vi "FipsAdjacent.vi"() -> (11 "Fips":i32[](array[numeric]))   [LabVIEW 2017] (continued)
\t\"Yukon-Koyukuk Census Area, AK\"\t02290\n\"Apache County, AZ\"\t04001\t\"Apache County, AZ\"\t04001\n\"Apache County, AZ\"\t04001\t\"Graham County, AZ\"\t04009\n\"Apache County, AZ\"\t04001\t\"Greenlee County, AZ\"\t04011\n\"Apache County, AZ\"\t04001\t\"Navajo County, AZ\"\t04017\n\"Apache County, AZ\"\t04001\t\"Montezuma County, CO\"\t08083\n\"Apache County, AZ\"\t04001\t\"Catron County, NM\"\t35003\n\"Apache County, AZ\"\t04001\t\"Cibola County, NM\"\t35006\n\"Apache County, AZ\"\t04001\t\"McKinley County, NM\"\t35031\n\"Apache County, AZ\"\t04001\t\"San Juan County, NM\"\t35045\n\"Apache County, AZ\"\t04001\t\"San Juan County, UT\"\t49037\n\"Cochise County, AZ\"\t04003\t\"Cochise County, AZ\"\t04003\n\"Cochise County, AZ\"\t04003\t\"Graham County, AZ\"\t04009\n\"Cochise County, AZ\"\t04003\t\"Greenlee County, AZ\"\t04011\n\"Cochise County, AZ\"\t04003\t\"Pima County, AZ\"\t04019\n\"Cochise County, AZ\"\t04003\t\"Santa Cruz County, AZ\"\t04023\n\"Cochise County, AZ\"\t04003\t\"Hidalgo County, NM\"\t35023\n\"Coconino County, AZ\"\t04005\t\"Coconino County, AZ\"\t04005\n\"Coconino County, AZ\"\t04005\t\"Gila County, AZ\"\t04007\n\"Coconino County, AZ\"\t04005\t\"Mohave County, AZ\"\t04015\n\"Coconino County, AZ\"\t04005\t\"Navajo County, AZ\"\t04017\n\"Coconino County, AZ\"\t04005\t\"Yavapai County, AZ\"\t04025\n\"Coconino County, AZ\"\t04005\t\"Kane County, UT\"\t49025\n\"Coconino County, AZ\"\t04005\t\"San Juan County, UT\"\t49037\n\"Gila County, AZ\"\t04007\t\"Coconino County, AZ\"\t04005\n\"Gila County, AZ\"\t04007\t\"Gila County, AZ\"\t04007\n\"Gila County, AZ\"\t04007\t\"Graham County, AZ\"\t04009\n\"Gila County, AZ\"\t04007\t\"Maricopa County, AZ\"\t04013\n\"Gila County, AZ\"\t04007\t\"Navajo County, AZ\"\t04017\n\"Gila County, AZ\"\t04007\t\"Pinal County, AZ\"\t04021\n\"Gila County, AZ\"\t04007\t\"Yavapai County, AZ\"\t04025\n\"Graham County, AZ\"\t04009\t\"Apache County, AZ\"\t04001\n\"Graham County, AZ\"\t04009\t\"Cochise County, AZ\"\t04003\n\"Graham County, AZ\"\t04009\t\"Gila County, AZ\"\t04007\n\"Graham County, AZ\"\t04009\t\"Graham County, AZ\"\t04009\n\"Graham County, AZ\"\t04009\t\"Greenlee County, AZ\"\t04011\n\"Graham County, AZ\"\t04009\t\"Navajo County, AZ\"\t04017\n\"Graham County, AZ\"\t04009\t\"Pima County, AZ\"\t04019\n\"Graham County, AZ\"\t04009\t\"Pinal County, AZ\"\t04021\n\"Greenlee County, AZ\"\t04011\t\"Apache County, AZ\"\t04001\n\"Greenlee County, AZ\"\t04011\t\"Cochise County, AZ\"\t04003\n\"Greenlee County, AZ\"\t04011\t\"Graham County, AZ\"\t04009\n\"Greenlee County, AZ\"\t04011\t\"Greenlee County, AZ\"\t04011\n\"Greenlee County, AZ\"\t04011\t\"Catron County, NM\"\t35003\n\"Greenlee County, AZ\"\t04011\t\"Grant County, NM\"\t35017\n\"Greenlee County, AZ\"\t04011\t\"Hidalgo County, NM\"\t35023\n\"La Paz County, AZ\"\t04012\t\"La Paz County, AZ\"\t04012\n\"La Paz County, AZ\"\t04012\t\"Maricopa County, AZ\"\t04013\n\"La Paz County, AZ\"\t04012\t\"Mohave County, AZ\"\t04015\n\"La Paz County, AZ\"\t04012\t\"Yavapai County, AZ\"\t04025\n\"La Paz County, AZ\"\t04012\t\"Yuma County, AZ\"\t04027\n\"La Paz County, AZ\"\t04012\t\"Imperial County, CA\"\t06025\n\"La Paz County, AZ\"\t04012\t\"Riverside County, CA\"\t06065\n\"La Paz County, AZ\"\t04012\t\"San Bernardino County, CA\"\t06071\n\"Maricopa County, AZ\"\t04013\t\"Gila County, AZ\"\t04007\n\"Maricopa County, AZ\"\t04013\t\"La Paz County, AZ\"\t04012\n\"Maricopa County, AZ\"\t04013\t\"Maricopa County, AZ\"\t04013\n\"Maricopa County, AZ\"\t04013\t\"Pima County, AZ\"\t04019\n\"Maricopa County, AZ\"\t04013\t\"Pinal County, AZ\"\t04021\n\"Maricopa County, AZ\"\t04013\t\"Yavapai County, AZ\"\t04025\n\"Maricopa County, AZ\"\t04013\t\"Yuma County, AZ\"\t04027\n\"Mohave County, AZ\"\t04015\t\"Coconino County, AZ\"\t04005\n\"Mohave County, AZ\"\t04015\t\"La Paz County, AZ\"\t04012\n\"Mohave County, AZ\"\t04015\t\"Mohave County, AZ\"\t04015\n\"Mohave County, AZ\"\t04015\t\"Yavapai County, AZ\"\t04025\n\"Mohave County, AZ\"\t04015\t\"San Bernardino County, CA\"\t06071\n\"Mohave County, AZ\"\t04015\t\"Clark County, NV\"\t32003\n\"Mohave County, AZ\"\t04015\t\"Lincoln County, NV\"\t32017\n\"Mohave County, AZ\"\t04015\t\"Kane County, UT\"\t49025\n\"Mohave County, AZ\"\t04015\t\"Washington County, UT\"\t49053\n\"Navajo County, AZ\"\t04017\t\"Apache County, AZ\"\t04001\n\"Navajo County, AZ\"\t04017\t\"Coconino County, AZ\"\t04005\n\"Navajo County, AZ\"\t04017\t\"Gila County, AZ\"\t04007\n\"Navajo County, AZ\"\t04017\t\"Graham County, AZ\"\t04009\n\"Navajo County, AZ\"\t04017\t\"Navajo County, AZ\"\t04017\n\"Navajo County, AZ\"\t04017\t\"San Juan County, UT\"\t49037\n\"Pima County, AZ\"\t04019\t\"Cochise County, AZ\"\t04003\n\"Pima County, AZ\"\t04019\t\"Graham County, AZ\"\t04009\n\"Pima County, AZ\"\t04019\t\"Maricopa County, AZ\"\t04013\n\"Pima County, AZ\"\t04019\t\"Pima County, AZ\"\t04019\n\"Pima County, AZ\"\t04019\t\"Pinal County, AZ\"\t04021\n\"Pima County, AZ\"\t04019\t\"Santa Cruz County, AZ\"\t04023\n\"Pima County, AZ\"\t04019\t\"Yuma County, AZ\"\t04027\n\"Pinal County, AZ\"\t04021\t\"Gila County, AZ\"\t04007\n\"Pinal County, AZ\"\t04021\t\"Graham County, AZ\"\t04009\n\"Pinal County, AZ\"\t04021\t\"Maricopa County, AZ\"\t04013\n\"Pinal County, AZ\"\t04021\t\"Pima County, AZ\"\t04019\n\"Pinal County, AZ\"\t04021\t\"Pinal County, AZ\"\t04021\n\"Santa Cruz County, AZ\"\t04023\t\"Cochise County, AZ\"\t04003\n\"Santa Cruz County, AZ\"\t04023\t\"Pima County, AZ\"\t04019\n\"Santa Cruz County, AZ\"\t04023\t\"Santa Cruz County, AZ\"\t04023\n\"Yavapai County, AZ\"\t04025\t\"Coconino County, AZ\"\t04005\n\"Yavapai County, AZ\"\t04025\t\"Gila County, AZ\"\t04007\n\"Yavapai County, AZ\"\t04025\t\"La Paz County, AZ\"\t04012\n\"Yavapai County, AZ\"\t04025\t\"Maricopa County, AZ\"\t04013\n\"Yavapai County, AZ\"\t04025\t\"Mohave County, AZ\"\t04015\n\"Yavapai County, AZ\"\t04025\t\"Yavapai County, AZ\"\t04025\n\"Yuma County, AZ\"\t04027\t\"La Paz County, AZ\"\t04012\n\"Yuma County, AZ\"\t04027\t\"Maricopa County, AZ\"\t04013\n\"Yuma County, AZ\"\t04027\t\"Pima County, AZ\"\t04019\n\"Yuma County, AZ\"\t04027\t\"Yuma County, AZ\"\t04027\n\"Yuma County, AZ\"\t04027\t\"Imperial County, CA\"\t06025\n\"Arkansas County, AR\"\t05001\t\"Arkansas County, AR\"\t05001\n\"Arkansas County, AR\"\t05001\t\"Desha County, AR\"\t05041\n\"Arkansas County, AR\"\t05001\t\"Jefferson County, AR\"\t05069\n\"Arkansas County, AR\"\t05001\t\"Lincoln County, AR\"\t05079\n\"Arkansas County, AR\"\t05001\t\"Lonoke County, AR\"\t05085\n\"Arkansas County, AR\"\t05001\t\"Monroe County, AR\"\t05095\n\"Arkansas County, AR\"\t05001\t\"Phillips County, AR\"\t05107\n\"Arkansas County, AR\"\t05001\t\"Prairie County, AR\"\t05117\n\"Ashley County, AR\"\t05003\t\"Ashley County, AR\"\t05003\n\"Ashley County, AR\"\t05003\t\"Bradley County, AR\"\t05011\n\"Ashley County, AR\"\t05003\t\"Chicot County, AR\"\t05017\n\"Ashley County, AR\"\t05003\t\"Drew County, AR\"\t05043\n\"Ashley County, AR\"\t05003\t\"Union County, AR\"\t05139\n\"Ashley County, AR\"\t05003\t\"Morehouse Parish, LA\"\t22067\n\"Ashley County, AR\"\t05003\t\"Union Parish, LA\"\t22111\n\"Baxter County, AR\"\t05005\t\"Baxter County, AR\"\t05005\n\"Baxter County, AR\"\t05005\t\"Fulton County, AR\"\t05049\n\"Baxter County, AR\"\t05005\t\"Izard County, AR\"\t05065\n\"Baxter County, AR\"\t05005\t\"Marion County, AR\"\t05089\n\"Baxter County, AR\"\t05005\t\"Searcy County, AR\"\t05129\n\"Baxter County, AR\"\t05005\t\"Stone County, AR\"\t05137\n\"Baxter County, AR\"\t05005\t\"Ozark County, MO\"\t29153\n\"Benton County, AR\"\t05007\t\"Benton County, AR\"\t05007\n\"Benton County, AR\"\t05007\t\"Carroll County, AR\"\t05015\n\"Benton County, AR\"\t05007\t\"Madison County, AR\"\t05087\n\"Benton County, AR\"\t05007\t\"Washington County, AR\"\t05143\n\"Benton County, AR\"\t05007\t\"Barry County, MO\"\t29009\n\"Benton County, AR\"\t05007\t\"McDonald County, MO\"\t29119\n\"Benton County, AR\"\t05007\t\"Adair County, OK\"\t40001\n\"Benton County, AR\"\t05007\t\"Delaware County, OK\"\t40041\n\"Boone County, AR\"\t05009\t\"Boone County, AR\"\t05009\n\"Boone County, AR\"\t05009\t\"Carroll County, AR\"\t05015\n\"Boone County, AR\"\t05009\t\"Marion County, AR\"\t05089\n\"Boone County, AR\"\t05009\t\"Newton County, AR\"\t05101\n\"Boone County, AR\"\t05009\t\"Searcy County, AR\"\t05129\n\"Boone County, AR\"\t05009\t\"Taney County, MO\"\t29213\n\"Bradley County, AR\"\t05011\t\"Ashley County, AR\"\t05003\n\"Bradley County, AR\"\t05011\t\"Bradley County, AR\"\t05011\n\"Bradley County, AR\"\t05011\t\"Calhoun County, AR\"\t05013\n\"Bradley County, AR\"\t05011\t\"Cleveland County, AR\"\t05025\n\"Bradley County, AR\"\t05011\t\"Drew County, AR\"\t05043\n\"Bradley County, AR\"\t05011\t\"Union County, AR\"\t05139\n\"Calhoun County, AR\"\t05013\t\"Bradley County, AR\"\t05011\n\"Calhoun County, AR\"\t05013\t\"Calhoun County, AR\"\t05013\n\"Calhoun County, AR\"\t05013\t\"Cleveland County, AR\"\t05025\n\"Calhoun County, AR\"\t05013\t\"Dallas County, AR\"\t05039\n\"Calhoun County, AR\"\t05013\t\"Ouachita County, AR\"\t05103\n\"Calhoun County, AR\"\t05013\t\"Union County, AR\"\t05139\n\"Carroll County, AR\"\t05015\t\"Benton County, AR\"\t05007\n\"Carroll County, AR\"\t05015\t\"Boone County, AR\"\t05009\n\"Carroll County, AR\"\t05015\t\"Carroll County, AR\"\t05015\n\"Carroll County, AR\"\t05015\t\"Madison County, AR\"\t05087\n\"Carroll County, AR\"\t05015\t\"Newton County, AR\"\t05101\n\"Carroll County, AR\"\t05015\t\"Barry County, MO\"\t29009\n\"Carroll County, AR\"\t05015\t\"Stone County, MO\"\t29209\n\"Carroll County, AR\"\t05015\t\"Taney County, MO\"\t29213\n\"Chicot County, AR\"\t05017\t\"Ashley County, AR\"\t05003\n\"Chicot County, AR\"\t05017\t\"Chicot County, AR\"\t05017\n\"Chicot County, AR\"\t05017\t\"Desha County, AR\"\t05041\n\"Chicot County, AR\"\t05017\t\"Drew County, AR\"\t05043\n\"Chicot County, AR\"\t05017\t\"East Carroll Parish, LA\"\t22035\n\"Chicot County, AR\"\t05017\t\"Morehouse Parish, LA\"\t22067\n\"Chicot County, AR\"\t05017\t\"West Carroll Parish, LA\"\t22123\n\"Chicot County, AR\"\t05017\t\"Bolivar County, MS\"\t28011\n\"Chicot County, AR\"\t05017\t\"Issaquena County, MS\"\t28055\n\"Chicot County, AR\"\t05017\t\"Washington County, MS\"\t28151\n\"Clark County, AR\"\t05019\t\"Clark County, AR\"\t05019\n\"Clark County, AR\"\t05019\t\"Dallas County, AR\"\t05039\n\"Clark County, AR\"\t05019\t\"Hot Spring County, AR\"\t05059\n\"Clark County, AR\"\t05019\t\"Montgomery County, AR\"\t05097\n\"Clark County, AR\"\t05019\t\"Nevada County, AR\"\t05099\n\"Clark County, AR\"\t05019\t\"Ouachita County, AR\"\t05103\n\"Clark County, AR\"\t05019\t\"Pike County, AR\"\t05109\n\"Clay County, AR\"\t05021\t\"Clay County, AR\"\t05021\n\"Clay County, AR\"\t05021\t\"Greene County, AR\"\t05055\n\"Clay County, AR\"\t05021\t\"Randolph County, AR\"\t05121\n\"Clay County, AR\"\t05021\t\"Butler County, MO\"\t29023\n\"Clay County, AR\"\t05021\t\"Dunklin County, MO\"\t29069\n\"Clay County, AR\"\t05021\t\"Ripley County, MO\"\t29181\n\"Cleburne County, AR\"\t05023\t\"Cleburne County, AR\"\t05023\n\"Cleburne County, AR\"\t05023\t\"Faulkner County, AR\"\t05045\n\"Cleburne County, AR\"\t05023\t\"Independence County, AR\"\t05063\n\"Cleburne County, AR\"\t05023\t\"Stone County, AR\"\t05137\n\"Cleburne County, AR\"\t05023\t\"Van Buren County, AR\"\t05141\n\"Cleburne County, AR\"\t05023\t\"White County, AR\"\t05145\n\"Cleveland County, AR\"\t05025\t\"Bradley County, AR\"\t05011\n\"Cleveland County, AR\"\t05025\t\"Calhoun County, AR\"\t05013\n\"Cleveland County, AR\"\t05025\t\"Cleveland County, AR\"\t05025\n\"Cleveland County, AR\"\t05025\t\"Dallas County, AR\"\t05039\n\"Cleveland County, AR\"\t05025\t\"Drew County, AR\"\t05043\n\"Cleveland County, AR\"\t05025\t\"Grant County, AR\"\t05053\n\"Cleveland County, AR\"\t05025\t\"Jefferson County, AR\"\t05069\n\"Cleveland County, AR\"\t05025\t\"Lincoln County, AR\"\t05079\n\"Columbia County, AR\"\t05027\t\"Columbia County, AR\"\t05027\n\"Columbia County, AR\"\t05027\t\"Lafayette County, AR\"\t05073\n\"Columbia County, AR\"\t05027\t\"Nevada County, AR\"\t05099\n\"Columbia County, AR\"\t05027\t\"Ouachita County, AR\"\t05103\n\"Columbia County, AR\"\t05027\t\"Union County, AR\"\t05139\n\"Columbia County, AR\"\t05027\t\"Claiborne Parish, LA\"\t22027\n\"Columbia County, AR\"\t05027\t\"Webster Parish, LA\"\t22119\n\"Conway County, AR\"\t05029\t\"Conway County, AR\"\t05029\n\"Conway County, AR\"\t05029\t\"Faulkner County, AR\"\t05045\n\"Conway County, AR\"\t05029\t\"Perry County, AR\"\t05105\n\"Conway County, AR\"\t05029\t\"Pope County, AR\"\t05115\n\"Conway County, AR\"\t05029\t\"Van Buren County, AR\"\t05141\n\"Conway County, AR\"\t05029\t\"Yell County, AR\"\t05149\n\"Craighead County, AR\"\t05031\t\"Craighead County, AR\"\t05031\n\"Craighead County, AR\"\t05031\t\"Greene County, AR\"\t05055\n\"Craighead County, AR\"\t05031\t\"Jackson County, AR\"\t05067\n\"Craighead County, AR\"\t05031\t\"Lawrence County, AR\"\t05075\n\"Craighead County, AR\"\t05031\t\"Mississippi County, AR\"\t05093\n\"Craighead County, AR\"\t05031\t\"Poinsett County, AR\"\t05111\n\"Craighead County, AR\"\t05031\t\"Dunklin County, MO\"\t29069\n\"Crawford County, AR\"\t05033\t\"Crawford County, AR\"\t05033\n\"Crawford County, AR\"\t05033\t\"Franklin County, AR\"\t05047\n\"Crawford County, AR\"\t05033\t\"Madison County, AR\"\t05087\n\"Crawford County, AR\"\t05033\t\"Sebastian County, AR\"\t05131\n\"Crawford County, AR\"\t05033\t\"Washington County, AR\"\t05143\n\"Crawford County, AR\"\t05033\t\"Adair County, OK\"\t40001\n\"Crawford County, AR\"\t05033\t\"Sequoyah County, OK\"\t40135\n\"Crittenden County, AR\"\t05035\t\"Crittenden County, AR\"\t05035\n\"Crittenden County, AR\"\t05035\t\"Cross County, AR\"\t05037\n\"Crittenden County, AR\"\t05035\t\"Lee County, AR\"\t05077\n\"Crittenden County, AR\"\t05035\t\"Mississippi County, AR\"\t05093\n\"Crittenden County, AR\"\t05035\t\"Poinsett County, AR\"\t05111\n\"Crittenden County, AR\"\t05035\t\"St. Francis County, AR\"\t05123\n\"Crittenden County, AR\"\t05035\t\"DeSoto County, MS\"\t28033\n\"Crittenden County, AR\"\t05035\t\"Tunica County, MS\"\t28143\n\"Crittenden County, AR\"\t05035\t\"Shelby County, TN\"\t47157\n\"Crittenden County, AR\"\t05035\t\"Tipton County, TN\"\t47167\n\"Cross County, AR\"\t05037\t\"Crittenden County, AR\"\t05035\n\"Cross County, AR\"\t05037\t\"Cross County, AR\"\t05037\n\"Cross County, AR\"\t05037\t\"Jackson County, AR\"\t05067\n\"Cross County, AR\"\t05037\t\"Poinsett County, AR\"\t05111\n\"Cross County, AR\"\t05037\t\"St. Francis County, AR\"\t05123\n\"Cross County, AR\"\t05037\t\"Woodruff County, AR\"\t05147\n\"Dallas County, AR\"\t05039\t\"Calhoun County, AR\"\t05013\n\"Dallas County, AR\"\t05039\t\"Clark County, AR\"\t05019\n\"Dallas County, AR\"\t05039\t\"Cleveland County, AR\"\t05025\n\"Dallas County, AR\"\t05039\t\"Dallas County, AR\"\t05039\n\"Dallas County, AR\"\t05039\t\"Grant County, AR\"\t05053\n\"Dallas County, AR\"\t05039\t\"Hot Spring County, AR\"\t05059\n\"Dallas County, AR\"\t05039\t\"Ouachita County, AR\"\t05103\n\"Desha County, AR\"\t05041\t\"Arkansas County, AR\"\t05001\n\"Desha County, AR\"\t05041\t\"Chicot County, AR\"\t05017\n\"Desha County, AR\"\t05041\t\"Desha County, AR\"\t05041\n\"Desha County, AR\"\t05041\t\"Drew County, AR\"\t05043\n\"Desha County, AR\"\t05041\t\"Lincoln County, AR\"\t05079\n\"Desha County, AR\"\t05041\t\"Phillips County, AR\"\t05107\n\"Desha County, AR\"\t05041\t\"Bolivar County, MS\"\t28011\n\"Drew County, AR\"\t05043\t\"Ashley County, AR\"\t05003\n\"Drew County, AR\"\t05043\t\"Bradley County, AR\"\t05011\n\"Drew County, AR\"\t05043\t\"Chicot County, AR\"\t05017\n\"Drew County, AR\"\t05043\t\"Cleveland County, AR\"\t05025\n\"Drew County, AR\"\t05043\t\"Desha County, AR\"\t05041\n\"Drew County, AR\"\t05043\t\"Drew County, AR\"\t05043\n\"Drew County, AR\"\t05043\t\"Lincoln County, AR\"\t05079\n\"Faulkner County, AR\"\t05045\t\"Cleburne County, AR\"\t05023\n\"Faulkner County, AR\"\t05045\t\"Conway County, AR\"\t05029\n\"Faulkner County, AR\"\t05045\t\"Faulkner County, AR\"\t05045\n\"Faulkner County, AR\"\t05045\t\"Lonoke County, AR\"\t05085\n\"Faulkner County, AR\"\t05045\t\"Perry County, AR\"\t05105\n\"Faulkner County, AR\"\t05045\t\"Pulaski County, AR\"\t05119\n\"Faulkner County, AR\"\t05045\t\"Van Buren County, AR\"\t05141\n\"Faulkner County, AR\"\t05045\t\"White County, AR\"\t05145\n\"Franklin County, AR\"\t05047\t\"Crawford County, AR\"\t05033\n\"Franklin County, AR\"\t05047\t\"Franklin County, AR\"\t05047\n\"Franklin County, AR\"\t05047\t\"Johnson County, AR\"\t05071\n\"Franklin County, AR\"\t05047\t\"Logan County, AR\"\t05083\n\"Franklin County, AR\"\t05047\t\"Madison County, AR\"\t05087\n\"Franklin County, AR\"\t05047\t\"Sebastian County, AR\"\t05131\n\"Fulton County, AR\"\t05049\t\"Baxter County, AR\"\t05005\n\"Fulton County, AR\"\t05049\t\"Fulton County, AR\"\t05049\n\"Fulton County, AR\"\t05049\t\"Izard County, AR\"\t05065\n\"Fulton County, AR\"\t05049\t\"Sharp County, AR\"\t05135\n\"Fulton County, AR\"\t05049\t\"Howell County, MO\"\t29091\n\"Fulton County, AR\"\t05049\t\"Oregon County, MO\"\t29149\n\"Fulton County, AR\"\t05049\t\"Ozark County, MO\"\t29153\n\"Garland County, AR\"\t05051\t\"Garland County, AR\"\t05051\n\"Garland County, AR\"\t05051\t\"Hot Spring County, AR\"\t05059\n\"Garland County, AR\"\t05051\t\"Montgomery County, AR\"\t05097\n\"Garland County, AR\"\t05051\t\"Perry County, AR\"\t05105\n\"Garland County, AR\"\t05051\t\"Saline County, AR\"\t05125\n\"Garland County, AR\"\t05051\t\"Yell County, AR\"\t05149\n\"Grant County, AR\"\t05053\t\"Cleveland County, AR\"\t05025\n\"Grant County, AR\"\t05053\t\"Dallas County, AR\"\t05039\n\"Grant County, AR\"\t05053\t\"Grant County, AR\"\t05053\n\"Grant County, AR\"\t05053\t\"Hot Spring County, AR\"\t05059\n\"Grant County, AR\"\t05053\t\"Jefferson County, AR\"\t05069\n\"Grant County, AR\"\t05053\t\"Pulaski County, AR\"\t05119\n\"Grant County, AR\"\t05053\t\"Saline County, AR\"\t05125\n\"Greene County, AR\"\t05055\t\"Clay County, AR\"\t05021\n\"Greene County, AR\"\t05055\t\"Craighead County, AR\"\t05031\n\"Greene County, AR\"\t05055\t\"Greene County, AR\"\t05055\n\"Greene County, AR\"\t05055\t\"Lawrence County, AR\"\t05075\n\"Greene County, AR\"\t05055\t\"Randolph County, AR\"\t05121\n\"Greene County, AR\"\t05055\t\"Dunklin County, MO\"\t29069\n\"Hempstead County, AR\"\t05057\t\"Hempstead County, AR\"\t05057\n\"Hempstead County, AR\"\t05057\t\"Howard County, AR\"\t05061\n\"Hempstead County, AR\"\t05057\t\"Lafayette County, AR\"\t05073\n\"Hempstead County, AR\"\t05057\t\"Little River County, AR\"\t05081\n\"Hempstead County, AR\"\t05057\t\"Miller County, AR\"\t05091\n\"Hempstead County, AR\"\t05057\t\"Nevada County, AR\"\t05099\n\"Hempstead County, AR\"\t05057\t\"Pike County, AR\"\t05109\n\"Hot Spring County, AR\"\t05059\t\"Clark County, AR\"\t05019\n\"Hot Spring County, AR\"\t05059\t\"Dallas County, AR\"\t05039\n\"Hot Spring County, AR\"\t05059\t\"Garland County, AR\"\t05051\n\"Hot Spring County, AR\"\t05059\t\"Grant County, AR\"\t05053\n\"Hot Spring County, AR\"\t05059\t\"Hot Spring County, AR\"\t05059\n\"Hot Spring County, AR\"\t05059\t\"Montgomery County, AR\"\t05097\n\"Hot Spring County, AR\"\t05059\t\"Saline County, AR\"\t05125\n\"Howard County, AR\"\t05061\t\"Hempstead County, AR\"\t05057\n\"Howard County, AR\"\t05061\t\"Howard County, AR\"\t05061\n\"Howard County, AR\"\t05061\t\"Little River County, AR\"\t05081\n\"Howard County, AR\"\t05061\t\"Montgomery County, AR\"\t05097\n\"Howard County, AR\"\t05061\t\"Pike County, AR\"\t05109\n\"Howard County, AR\"\t05061\t\"Polk County, AR\"\t05113\n\"Howard County, AR\"\t05061\t\"Sevier County, AR\"\t05133\n\"Independence County, AR\"\t05063\t\"Cleburne County, AR\"\t05023\n\"Independence County, AR\"\t05063\t\"Independence County, AR\"\t05063\n\"Independence County, AR\"\t05063\t\"Izard County, AR\"\t05065\n\"Independence County, AR\"\t05063\t\"Jackson County, AR\"\t05067\n\"Independence County, AR\"\t05063\t\"Lawrence County, AR\"\t05075\n\"Independence County, AR\"\t05063\t\"Sharp County, AR\"\t05135\n\"Independence County, AR\"\t05063\t\"Stone County, AR\"\t05137\n\"Independence County, AR\"\t05063\t\"White County, AR\"\t05145\n\"Izard County, AR\"\t05065\t\"Baxter County, AR\"\t05005\n\"Izard County, AR\"\t05065\t\"Fulton County, AR\"\t05049\n\"Izard County, AR\"\t05065\t\"Independence County, AR\"\t05063\n\"Izard County, AR\"\t05065\t\"Izard County, AR\"\t05065\n\"Izard County, AR\"\t05065\t\"Sharp County, AR\"\t05135\n\"Izard County, AR\"\t05065\t\"Stone County, AR\"\t05137\n\"Jackson County, AR\"\t05067\t\"Craighead County, AR\"\t05031\n\"Jackson County, AR\"\t05067\t\"Cross County, AR\"\t05037\n\"Jackson County, AR\"\t05067\t\"Independence County, AR\"\t05063\n\"Jackson County, AR\"\t05067\t\"Jackson County, AR\"\t05067\n\"Jackson County, AR\"\t05067\t\"Lawrence County, AR\"\t05075\n\"Jackson County, AR\"\t05067\t\"Poinsett County, AR\"\t05111\n\"Jackson County, AR\"\t05067\t\"White County, AR\"\t05145\n\"Jackson County, AR\"\t05067\t\"Woodruff County, AR\"\t05147\n\"Jefferson County, AR\"\t05069\t\"Arkansas County, AR\"\t05001\n\"Jefferson County, AR\"\t05069\t\"Cleveland County, AR\"\t05025\n\"Jefferson County, AR\"\t05069\t\"Grant County, AR\"\t05053\n\"Jefferson County, AR\"\t05069\t\"Jefferson County, AR\"\t05069\n\"Jefferson County, AR\"\t05069\t\"Lincoln County, AR\"\t05079\n\"Jefferson County, AR\"\t05069\t\"Lonoke County, AR\"\t05085\n\"Jefferson County, AR\"\t05069\t\"Pulaski County, AR\"\t05119\n\"Johnson County, AR\"\t05071\t\"Franklin County, AR\"\t05047\n\"Johnson County, AR\"\t05071\t\"Johnson County, AR\"\t05071\n\"Johnson County, AR\"\t05071\t\"Logan County, AR\"\t05083\n\"Johnson County, AR\"\t05071\t\"Madison County, AR\"\t05087\n\"Johnson County, AR\"\t05071\t\"Newton County, AR\"\t05101\n\"Johnson County, AR\"\t05071\t\"Pope County, AR\"\t05115\n\"Lafayette County, AR\"\t05073\t\"Columbia County, AR\"\t05027\n\"Lafayette County, AR\"\t05073\t\"Hempstead County, AR\"\t05057\n\"Lafayette County, AR\"\t05073\t\"Lafayette County, AR\"\t05073\n\"Lafayette County, AR\"\t05073\t\"Miller County, AR\"\t05091\n\"Lafayette County, AR\"\t05073\t\"Nevada County, AR\"\t05099\n\"Lafayette County, AR\"\t05073\t\"Bossier Parish, LA\"\t22015\n\"Lafayette County, AR\"\t05073\t\"Webster Parish, LA\"\t22119\n\"Lawrence County, AR\"\t05075\t\"Craighead County, AR\"\t05031\n\"Lawrence County, AR\"\t05075\t\"Greene County, AR\"\t05055\n\"Lawrence County, AR\"\t05075\t\"Independence County, AR\"\t05063\n\"Lawrence County, AR\"\t05075\t\"Jackson County, AR\"\t05067\n\"Lawrence County, AR\"\t05075\t\"Lawrence County, AR\"\t05075\n\"Lawrence County, AR\"\t05075\t\"Randolph County, AR\"\t05121\n\"Lawrence County, AR\"\t05075\t\"Sharp County, AR\"\t05135\n\"Lee County, AR\"\t05077\t\"Crittenden County, AR\"\t05035\n\"Lee County, AR\"\t05077\t\"Lee County, AR\"\t05077\n\"Lee County, AR\"\t05077\t\"Monroe County, AR\"\t05095\n\"Lee County, AR\"\t05077\t\"Phillips County, AR\"\t05107\n\"Lee County, AR\"\t05077\t\"St. Francis County, AR\"\t05123\n\"Lee County, AR\"\t05077\t\"Tunica County, MS\"\t28143\n\"Lincoln County, AR\"\t05079\t\"Arkansas County, AR\"\t05001\n\"Lincoln County, AR\"\t05079\t\"Cleveland County, AR\"\t05025\n\"Lincoln County, AR\"\t05079\t\"Desha County, AR\"\t05041\n\"Lincoln County, AR\"\t05079\t\"Drew County, AR\"\t05043\n\"Lincoln County, AR\"\t05079\t\"Jefferson County, AR\"\t05069\n\"Lincoln County, AR\"\t05079\t\"Lincoln County, AR\"\t05079\n\"Little River County, AR\"\t05081\t\"Hempstead County, AR\"\t05057\n\"Little River County, AR\"\t05081\t\"Howard County, AR\"\t05061\n\"Little River County, AR\"\t05081\t\"Little River County, AR\"\t05081\n\"Little River County, AR\"\t05081\t\"Miller County, AR\"\t05091\n\"Little River County, AR\"\t05081\t\"Sevier County, AR\"\t05133\n\"Little River County, AR\"\t05081\t\"McCurtain County, OK\"\t40089\n\"Little River County, AR\"\t05081\t\"Bowie County, TX\"\t48037\n\"Logan County, AR\"\t05083\t\"Franklin County, AR\"\t05047\n\"Logan County, AR\"\t05083\t\"Johnson County, AR\"\t05071\n\"Logan County, AR\"\t05083\t\"Logan County, AR\"\t05083\n\"Logan County, AR\"\t05083\t\"Pope County, AR\"\t05115\n\"Logan County, AR\"\t05083\t\"Scott County, AR\"\t05127\n\"Logan County, AR\"\t05083\t\"Sebastian County, AR\"\t05131\n\"Logan County, AR\"\t05083\t\"Yell County, AR\"\t05149\n\"Lonoke County, AR\"\t05085\t\"Arkansas County, AR\"\t05001\n\"Lonoke County, AR\"\t05085\t\"Faulkner County, AR\"\t05045\n\"Lonoke County, AR\"\t05085\t\"Jefferson County, AR\"\t05069\n\"Lonoke County, AR\"\t05085\t\"Lonoke County, AR\"\t05085\n\"Lonoke County, AR\"\t05085\t\"Prairie County, AR\"\t05117\n\"Lonoke County, AR\"\t05085\t\"Pulaski County, AR\"\t05119\n\"Lonoke County, AR\"\t05085\t\"White County, AR\"\t05145\n\"Madison County, AR\"\t05087\t\"Benton County, AR\"\t05007\n\"Madison County, AR\"\t05087\t\"Carroll County, AR\"\t05015\n\"Madison County, AR\"\t05087\t\"Crawford County, AR\"\t05033\n\"Madison County, AR\"\t05087\t\"Franklin County, AR\"\t05047\n\"Madison County, AR\"\t05087\t\"Johnson County, AR\"\t05071\n\"Madison County, AR\"\t05087\t\"Madison County, AR\"\t05087\n\"Madison County, AR\"\t05087\t\"Newton County, AR\"\t05101\n\"Madison County, AR\"\t05087\t\"Washington County, AR\"\t05143\n\"Marion County, AR\"\t05089\t\"Baxter County, AR\"\t05005\n\"Marion County, AR\"\t05089\t\"Boone County, AR\"\t05009\n\"Marion County, AR\"\t05089\t\"Marion County, AR\"\t05089\n\"Marion County, AR\"\t05089\t\"Searcy County, AR\"\t05129\n\"Marion County, AR\"\t05089\t\"Ozark County, MO\"\t29153\n\"Marion County, AR\"\t05089\t\"Taney County, MO\"\t29213\n\"Miller County, AR\"\t05091\t\"Hempstead County, AR\"\t05057\n\"Miller County, AR\"\t05091\t\"Lafayette County, AR\"\t05073\n\"Miller County, AR\"\t05091\t\"Little River County, AR\"\t05081\n\"Miller County, AR\"\t05091\t\"Miller County, AR\"\t05091\n\"Miller County, AR\"\t05091\t\"Bossier Parish, LA\"\t22015\n\"Miller County, AR\"\t05091\t\"Caddo Parish, LA\"\t22017\n\"Miller County, AR\"\t05091\t\"Bowie County, TX\"\t48037\n\"Miller County, AR\"\t05091\t\"Cass County, TX\"\t48067\n\"Mississippi County, AR\"\t05093\t\"Craighead County, AR\"\t05031\n\"Mississippi County, AR\"\t05093\t\"Crittenden County, AR\"\t05035\n\"Mississippi County, AR\"\t05093\t\"Mississippi County, AR\"\t05093\n\"Mississippi County, AR\"\t05093\t\"Poinsett County, AR\"\t05111\n\"Mississippi County, AR\"\t05093\t\"Dunklin County, MO\"\t29069\n\"Mississippi County, AR\"\t05093\t\"Pemiscot County, MO\"\t29155\n\"Mississippi County, AR\"\t05093\t\"Dyer County, TN\"\t47045\n\"Mississippi County, AR\"\t05093\t\"Lauderdale County, TN\"\t47097\n\"Mississippi County, AR\"\t05093\t\"Shelby County, TN\"\t47157\n\"Mississippi County, AR\"\t05093\t\"Tipton County, TN\"\t47167\n\"Monroe County, AR\"\t05095\t\"Arkansas County, AR\"\t05001\n\"Monroe County, AR\"\t05095\t\"Lee County, AR\"\t05077\n\"Monroe County, AR\"\t05095\t\"Monroe County, AR\"\t05095\n\"Monroe County, AR\"\t05095\t\"Phillips County, AR\"\t05107\n\"Monroe County, AR\"\t05095\t\"Prairie County, AR\"\t05117\n\"Monroe County, AR\"\t05095\t\"St. Francis County, AR\"\t05123\n\"Monroe County, AR\"\t05095\t\"Woodruff County, AR\"\t05147\n\"Montgomery County, AR\"\t05097\t\"Clark County, AR\"\t05019\n\"Montgomery County, AR\"\t05097\t\"Garland County, AR\"\t05051\n\"Montgomery County, AR\"\t05097\t\"Hot Spring County, AR\"\t05059\n\"Montgomery County, AR\"\t05097\t\"Howard County, AR\"\t05061\n\"Montgomery County, AR\"\t05097\t\"Montgomery County, AR\"\t05097\n\"Montgomery County, AR\"\t05097\t\"Pike County, AR\"\t05109\n\"Montgomery County, AR\"\t05097\t\"Polk County, AR\"\t05113\n\"Montgomery County, AR\"\t05097\t\"Scott County, AR\"\t05127\n\"Montgomery County, AR\"\t05097\t\"Yell County, AR\"\t05149\n\"Nevada County, AR\"\t05099\t\"Clark County, AR\"\t05019\n\"Nevada County, AR\"\t05099\t\"Columbia County, AR\"\t05027\n\"Nevada County, AR\"\t05099\t\"Hempstead County, AR\"\t05057\n\"Nevada County, AR\"\t05099\t\"Lafayette County, AR\"\t05073\n\"Nevada County, AR\"\t05099\t\"Nevada County, AR\"\t05099\n\"Nevada County, AR\"\t05099\t\"Ouachita County, AR\"\t05103\n\"Nevada County, AR\"\t05099\t\"Pike County, AR\"\t05109\n\"Newton County, AR\"\t05101\t\"Boone County, AR\"\t05009\n\"Newton County, AR\"\t05101\t\"Carroll County, AR\"\t05015\n\"Newton County, AR\"\t05101\t\"Johnson County, AR\"\t05071\n\"Newton County, AR\"\t05101\t\"Madison County, AR\"\t05087\n\"Newton County, AR\"\t05101\t\"Newton County, AR\"\t05101\n\"Newton County, AR\"\t05101\t\"Pope County, AR\"\t05115\n\"Newton County, AR\"\t05101\t\"Searcy County, AR\"\t05129\n\"Ouachita County, AR\"\t05103\t\"Calhoun County, AR\"\t05013\n\"Ouachita County, AR\"\t05103\t\"Clark County, AR\"\t05019\n\"Ouachita County, AR\"\t05103\t\"Columbia County, AR\"\t05027\n\"Ouachita County, AR\"\t05103\t\"Dallas County, AR\"\t05039\n\"Ouachita County, AR\"\t05103\t\"Nevada County, AR\"\t05099\n\"Ouachita County, AR\"\t05103\t\"Ouachita County, AR\"\t05103\n\"Ouachita County, AR\"\t05103\t\"Union County, AR\"\t05139\n\"Perry County, AR\"\t05105\t\"Conway County, AR\"\t05029\n\"Perry County, AR\"\t05105\t\"Faulkner County, AR\"\t05045\n\"Perry County, AR\"\t05105\t\"Garland County, AR\"\t05051\n\"Perry County, AR\"\t05105\t\"Perry County, AR\"\t05105\n\"Perry County, AR\"\t05105\t\"Pulaski County, AR\"\t05119\n\"Perry County, AR\"\t05105\t\"Saline County, AR\"\t05125\n\"Perry County, AR\"\t05105\t\"Yell County, AR\"\t05149\n\"Phillips County, AR\"\t05107\t\"Arkansas County, AR\"\t05001\n\"Phillips County, AR\"\t05107\t\"Desha County, AR\"\t05041\n\"Phillips County, AR\"\t05107\t\"Lee County, AR\"\t05077\n\"Phillips County, AR\"\t05107\t\"Monroe County, AR\"\t05095\n\"Phillips County, AR\"\t05107\t\"Phillips County, AR\"\t05107\n\"Phillips County, AR\"\t05107\t\"Bolivar County, MS\"\t28011\n\"Phillips County, AR\"\t05107\t\"Coahoma County, MS\"\t28027\n\"Phillips County, AR\"\t05107\t\"Tunica County, MS\"\t28143\n\"Pike County, AR\"\t05109\t\"Clark County, AR\"\t05019\n\"Pike County, AR\"\t05109\t\"Hempstead County, AR\"\t05057\n\"Pike County, AR\"\t05109\t\"Howard County, AR\"\t05061\n\"Pike County, AR\"\t05109\t\"Montgomery County, AR\"\t05097\n\"Pike County, AR\"\t05109\t\"Nevada County, AR\"\t05099\n\"Pike County, AR\"\t05109\t\"Pike County, AR\"\t05109\n\"Pike County, AR\"\t05109\t\"Polk County, AR\"\t05113\n\"Poinsett County, AR\"\t05111\t\"Craighead County, AR\"\t05031\n\"Poinsett County, AR\"\t05111\t\"Crittenden County, AR\"\t05035\n\"Poinsett County, AR\"\t05111\t\"Cross County, AR\"\t05037\n\"Poinsett County, AR\"\t05111\t\"Jackson County, AR\"\t05067\n\"Poinsett County, AR\"\t05111\t\"Mississippi County, AR\"\t05093\n\"Poinsett County, AR\"\t05111\t\"Poinsett County, AR\"\t05111\n\"Polk County, AR\"\t05113\t\"Howard County, AR\"\t05061\n\"Polk County, AR\"\t05113\t\"Montgomery County, AR\"\t05097\n\"Polk County, AR\"\t05113\t\"Pike County, AR\"\t05109\n\"Polk County, AR\"\t05113\t\"Polk County, AR\"\t05113\n\"Polk County, AR\"\t05113\t\"Scott County, AR\"\t05127\n\"Polk County, AR\"\t05113\t\"Sevier County, AR\"\t05133\n\"Polk County, AR\"\t05113\t\"Le Flore County, OK\"\t40079\n\"Polk County, AR\"\t05113\t\"McCurtain County, OK\"\t40089\n\"Pope County, AR\"\t05115\t\"Conway County, AR\"\t05029\n\"Pope County, AR\"\t05115\t\"Johnson County, AR\"\t05071\n\"Pope County, AR\"\t05115\t\"Logan County, AR\"\t05083\n\"Pope County, AR\"\t05115\t\"Newton County, AR\"\t05101\n\"Pope County, AR\"\t05115\t\"Pope County, AR\"\t05115\n\"Pope County, AR\"\t05115\t\"Searcy County, AR\"\t05129\n\"Pope County, AR\"\t05115\t\"Van Buren County, AR\"\t05141\n\"Pope County, AR\"\t05115\t\"Yell County, AR\"\t05149\n\"Prairie County, AR\"\t05117\t\"Arkansas County, AR\"\t05001\n\"Prairie County, AR\"\t05117\t\"Lonoke County, AR\"\t05085\n\"Prairie County, AR\"\t05117\t\"Monroe County, AR\"\t05095\n\"Prairie County, AR\"\t05117\t\"Prairie County, AR\"\t05117\n\"Prairie County, AR\"\t05117\t\"White County, AR\"\t05145\n\"Prairie County, AR\"\t05117\t\"Woodruff County, AR\"\t05147\n\"Pulaski County, AR\"\t05119\t\"Faulkner County, AR\"\t05045\n\"Pulaski County, AR\"\t05119\t\"Grant County, AR\"\t05053\n\"Pulaski County, AR\"\t05119\t\"Jefferson County, AR\"\t05069\n\"Pulaski County, AR\"\t05119\t\"Lonoke County, AR\"\t05085\n\"Pulaski County, AR\"\t05119\t\"Perry County, AR\"\t05105\n\"Pulaski County, AR\"\t05119\t\"Pulaski County, AR\"\t05119\n\"Pulaski County, AR\"\t05119\t\"Saline County, AR\"\t05125\n\"Randolph County, AR\"\t05121\t\"Clay County, AR\"\t05021\n\"Randolph County, AR\"\t05121\t\"Greene County, AR\"\t05055\n\"Randolph County, AR\"\t05121\t\"Lawrence County, AR\"\t05075\n\"Randolph County, AR\"\t05121\t\"Randolph County, AR\"\t05121\n\"Randolph County, AR\"\t05121\t\"Sharp County, AR\"\t05135\n\"Randolph County, AR\"\t05121\t\"Oregon County, MO\"\t29149\n\"Randolph County, AR\"\t05121\t\"Ripley County, MO\"\t29181\n\"St. Francis County, AR\"\t05123\t\"Crittenden County, AR\"\t05035\n\"St. Francis County, AR\"\t05123\t\"Cross County, AR\"\t05037\n\"St. Francis County, AR\"\t05123\t\"Lee County, AR\"\t05077\n\"St. Francis County, AR\"\t05123\t\"Monroe County, AR\"\t05095\n\"St. Francis County, AR\"\t05123\t\"St. Francis County, AR\"\t05123\n\"St. Francis County, AR\"\t05123\t\"Woodruff County, AR\"\t05147\n\"Saline County, AR\"\t05125\t\"Garland County, AR\"\t05051\n\"Saline County, AR\"\t05125\t\"Grant County, AR\"\t05053\n\"Saline County, AR\"\t05125\t\"Hot Spring County, AR\"\t05059\n\"Saline County, AR\"\t05125\t\"Perry County, AR\"\t05105\n\"Saline County, AR\"\t05125\t\"Pulaski County, AR\"\t05119\n\"Saline County, AR\"\t05125\t\"Saline County, AR\"\t05125\n\"Scott County, AR\"\t05127\t\"Logan County, AR\"\t05083\n\"Scott County, AR\"\t05127\t\"Montgomery County, AR\"\t05097\n\"Scott County, AR\"\t05127\t\"Polk County, AR\"\t05113\n\"Scott County, AR\"\t05127\t\"Scott County, AR\"\t05127\n\"Scott County, AR\"\t05127\t\"Sebastian County, AR\"\t05131\n\"Scott County, AR\"\t05127\t\"Yell County, AR\"\t05149\n\"Scott County, AR\"\t05127\t\"Le Flore County, OK\"\t40079\n\"Searcy County, AR\"\t05129\t\"Baxter County, AR\"\t05005\n\"Searcy County, AR\"\t05129\t\"Boone County, AR\"\t05009\n\"Searcy County, AR\"\t05129\t\"Marion County, AR\"\t05089\n\"Searcy County, AR\"\t05129\t\"Newton County, AR\"\t05101\n\"Searcy County, AR\"\t05129\t\"Pope County, AR\"\t05115\n\"Searcy County, AR\"\t05129\t\"Searcy County, AR\"\t05129\n\"Searcy County, AR\"\t05129\t\"Stone County, AR\"\t05137\n\"Searcy County, AR\"\t05129\t\"Van Buren County, AR\"\t05141\n\"Sebastian County, AR\"\t05131\t\"Crawford County, AR\"\t05033\n\"Sebastian County, AR\"\t05131\t\"Franklin County, AR\"\t05047\n\"Sebastian County, AR\"\t05131\t\"Logan County, AR\"\t05083\n\"Sebastian County, AR\"\t05131\t\"Scott County, AR\"\t05127\n\"Sebastian County, AR\"\t05131\t\"Sebastian County, AR\"\t05131\n\"Sebastian County, AR\"\t05131\t\"Le Flore County, OK\"\t40079\n\"Sebastian County, AR\"\t05131\t\"Sequoyah County, OK\"\t40135\n\"Sevier County, AR\"\t05133\t\"Howard County, AR\"\t05061\n\"Sevier County, AR\"\t05133\t\"Little River County, AR\"\t05081\n\"Sevier County, AR\"\t05133\t\"Polk County, AR\"\t05113\n\"Sevier County, AR\"\t05133\t\"Sevier County, AR\"\t05133\n\"Sevier County, AR\"\t05133\t\"McCurtain County, OK\"\t40089\n\"Sharp County, AR\"\t05135\t\"Fulton County, AR\"\t05049\n\"Sharp County, AR\"\t05135\t\"Independence County, AR\"\t05063\n\"Sharp County, AR\"\t05135\t\"Izard County, AR\"\t05065\n\"Sharp County, AR\"\t05135\t\"Lawrence County, AR\"\t05075\n\"Sharp County, AR\"\t05135\t\"Randolph County, AR\"\t05121\n\"Sharp County, AR\"\t05135\t\"Sharp County, AR\"\t05135\n\"Sharp County, AR\"\t05135\t\"Oregon County, MO\"\t29149\n\"Stone County, AR\"\t05137\t\"Baxter County, AR\"\t05005\n\"Stone County, AR\"\t05137\t\"Cleburne County, AR\"\t05023\n\"Stone County, AR\"\t05137\t\"Independence County, AR\"\t05063\n\"Stone County, AR\"\t05137\t\"Izard County, AR\"\t05065\n\"Stone County, AR\"\t05137\t\"Searcy County, AR\"\t05129\n\"Stone County, AR\"\t05137\t\"Stone County, AR\"\t05137\n\"Stone County, AR\"\t05137\t\"Van Buren County, AR\"\t05141\n\"Union County, AR\"\t05139\t\"Ashley County, AR\"\t05003\n\"Union County, AR\"\t05139\t\"Bradley County, AR\"\t05011\n\"Union County, AR\"\t05139\t\"Calhoun County, AR\"\t05013\n\"Union County, AR\"\t05139\t\"Columbia County, AR\"\t05027\n\"Union County, AR\"\t05139\t\"Ouachita County, AR\"\t05103\n\"Union County, AR\"\t05139\t\"Union County, AR\"\t05139\n\"Union County, AR\"\t05139\t\"Claiborne Parish, LA\"\t22027\n\"Union County, AR\"\t05139\t\"Morehouse Parish, LA\"\t22067\n\"Union County, AR\"\t05139\t\"Union Parish, LA\"\t22111\n\"Van Buren County, AR\"\t05141\t\"Cleburne County, AR\"\t05023\n\"Van Buren County, AR\"\t05141\t\"Conway County, AR\"\t05029\n\"Van Buren County, AR\"\t05141\t\"Faulkner County, AR\"\t05045\n\"Van Buren County, AR\"\t05141\t\"Pope County, AR\"\t05115\n\"Van Buren County, AR\"\t05141\t\"Searcy County, AR\"\t05129\n\"Van Buren County, AR\"\t05141\t\"Stone County, AR\"\t05137\n\"Van Buren County, AR\"\t05141\t\"Van Buren County, AR\"\t05141\n\"Washington County, AR\"\t05143\t\"Benton County, AR\"\t05007\n\"Washington County, AR\"\t05143\t\"Crawford County, AR\"\t05033\n\"Washington County, AR\"\t05143\t\"Madison County, AR\"\t05087\n\"Washington County, AR\"\t05143\t\"Washington County, AR\"\t05143\n\"Washington County, AR\"\t05143\t\"Adair County, OK\"\t40001\n\"White County, AR\"\t05145\t\"Cleburne County, AR\"\t05023\n\"White County, AR\"\t05145\t\"Faulkner County, AR\"\t05045\n\"White County, AR\"\t05145\t\"Independence County, AR\"\t05063\n\"White County, AR\"\t05145\t\"Jackson County, AR\"\t05067\n\"White County, AR\"\t05145\t\"Lonoke County, AR\"\t05085\n\"White County, AR\"\t05145\t\"Prairie County, AR\"\t05117\n\"White County, AR\"\t05145\t\"White County, AR\"\t05145\n\"White County, AR\"\t05145\t\"Woodruff County, AR\"\t05147\n\"Woodruff County, AR\"\t05147\t\"Cross County, AR\"\t05037\n\"Woodruff County, AR\"\t05147\t\"Jackson County, AR\"\t05067\n\"Woodruff County, AR\"\t05147\t\"Monroe County, AR\"\t05095\n\"Woodruff County, AR\"\t05147\t\"Prairie County, AR\"\t05117\n\"Woodruff County, AR\"\t05147\t\"St. Francis County, AR\"\t05123\n\"Woodruff County, AR\"\t05147\t\"White County, AR\"\t05145\n\"Woodruff County, AR\"\t05147\t\"Woodruff County, AR\"\t05147\n\"Yell County, AR\"\t05149\t\"Conway County, AR\"\t05029\n\"Yell County, AR\"\t05149\t\"Garland County, AR\"\t05051\n\"Yell County, AR\"\t05149\t\"Logan County, AR\"\t05083\n\"Yell County, AR\"\t05149\t\"Montgomery County, AR\"\t05097\n\"Yell County, AR\"\t05149\t\"Perry County, AR\"\t05105\n\"Yell County, AR\"\t05149\t\"Pope County, AR\"\t05115\n\"Yell County, AR\"\t05149\t\"Scott County, AR\"\t05127\n\"Yell County, AR\"\t05149\t\"Yell County, AR\"\t05149\n\"Alameda County, CA\"\t06001\t\"Alameda County, CA\"\t06001\n\"Alameda County, CA\"\t06001\t\"Contra Costa County, CA\"\t06013\n\"Alameda County, CA\"\t06001\t\"San Francisco County, CA\"\t06075\n\"Alameda County, CA\"\t06001\t\"San Joaquin County, CA\"\t06077\n\"Alameda County, CA\"\t06001\t\"San Mateo County, CA\"\t06081\n\"Alameda County, CA\"\t06001\t\"Santa Clara County, CA\"\t06085\n\"Alameda County, CA\"\t06001\t\"Stanislaus County, CA\"\t06099\n\"Alpine County, CA\"\t06003\t\"Alpine County, CA\"\t06003\n\"Alpine County, CA\"\t06003\t\"Amador County, CA\"\t06005\n\"Alpine County, CA\"\t06003\t\"Calaveras County, CA\"\t06009\n\"Alpine County, CA\"\t06003\t\"El Dorado County, CA\"\t06017\n\"Alpine County, CA\"\t06003\t\"Mono County, CA\"\t06051\n\"Alpine County, CA\"\t06003\t\"Tuolumne County, CA\"\t06109\n\"Alpine County, CA\"\t06003\t\"Douglas County, NV\"\t32005\n\"Amador County, CA\"\t06005\t\"Alpine County, CA\"\t06003\n\"Amador County, CA\"\t06005\t\"Amador County, CA\"\t06005\n\"Amador County, CA\"\t06005\t\"Calaveras County, CA\"\t06009\n\"Amador County, 
